vi "Get Status.vi"(8 "error in":errorcluster) -> (0 "error out":errorcluster, 3 "Messages":i32)   [LabVIEW 2025, in "CAN-LIN Raw Bus Capture.lvclass"]
uses:
  CAN-LIN Raw Bus Capture.lvclass
  CAN-LIN Raw Bus Capture.lvclass/CAN-LIN Raw Bus Capture.ctl
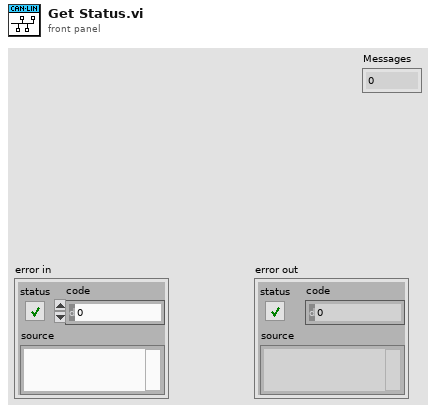
[diagram p1: front panel]
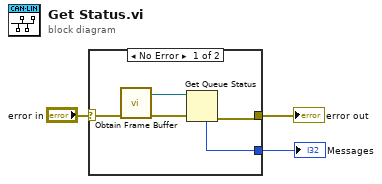
[diagram p0: block diagram]
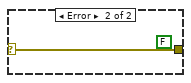
[diagram p2: hidden frame]
diagram:
  n1 = case shown="No Error" "error in" {
    selector: "error in" -> [w8 w9]
    tunnel: [w5 w9] -> w2
    tunnel: [w4 _] -> w1
    frame No Error {
      n2 = call "Obtain Frame Buffer.vi"("error in"=w8) -> ("error out"=w6:errorcluster, "queue out"=w7:refnum<queue>)  [unwired: 9 in]
      n3 = Get Queue Status(queue=w7, error in (no error)=w6) -> (error out=w5:errorcluster, # elements in queue=w4:i32)  [unwired: 1 in, 6 out]
    }
    frame Error {
      (unwired) FALSE ("overflow?")
    }
  }
  "error out" <- w2
  "Messages" <- w1
